vi "decodeBoolean.vi"(8 "error in (no error)":errorcluster, 10 "ByteArray":u8[](array[numeric])) -> (0 "error out":errorcluster, 1 "Boolean":bool, 2 "variant":variant, 3 "RemainingBytes":u8[](array[numeric]), 5 "Type":string)   [LabVIEW 2016, in "MsgPack.lvlib"]
uses:
  MsgPack.lvlib
  <vilib>/Utility/error.llb/Error Cluster From Error Code.vi
  <vilib>/ErrorRing/Error Ring.xnode
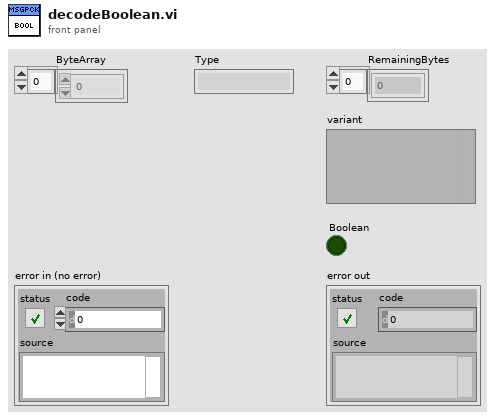
[diagram p1: front panel]
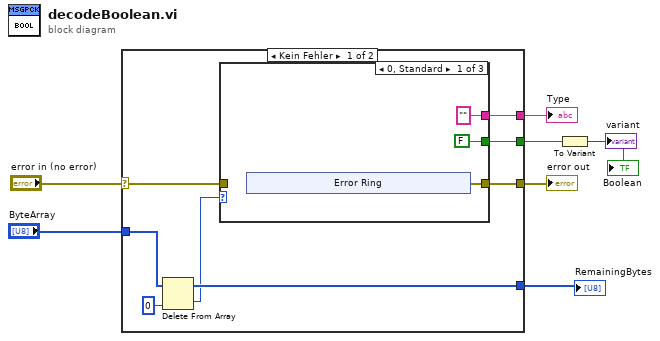
[diagram p0: block diagram]
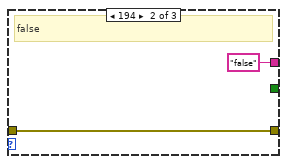
[diagram p2: hidden frame]
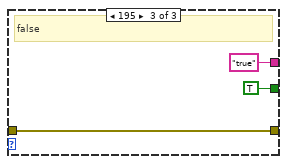
[diagram p3: hidden frame]
diagram:
  n1 = case shown="Kein Fehler" "error in (no error)" {
    selector: "error in (no error)" -> [w8 w30]
    tunnel: [w15 w30] -> w6
    tunnel: [w14 _] -> w5
    tunnel: [w13 _] -> w4
    tunnel: "ByteArray" -> [w12 w29]
    tunnel: [w11 w29] -> w2
    frame No Error {
      n2 = Delete From Array(array=w12, index=0) -> (deleted portion=w9:u8, array with subset deleted=w11:u8[])  [unwired: 1 in]
      n3 = case shown="0, Standard" w9 {
        tunnel: [w16 w25 w28] -> w15
        tunnel: w8 -> [_ w25 w28]
        tunnel: ["" "false" "true"] -> w14
        tunnel: [FALSE _ TRUE] -> w13
        frame 0, Default {
          n4 = xnode "Error Ring"() -> ("Fehler (Ausgang)"=w16:errorcluster)
        }
        frame 194 {
          # "false"
        }
        frame 195 {
          # "false"
        }
      }
    }
    frame Error {
    }
  }
  "error out" <- w6
  "Type" <- w5
  "Boolean" <- w4
  "RemainingBytes" <- w2
  n5 = To Variant(anything=w4) -> (Variant=→"variant":variant)
